vi "FP_Size Inside Bounds.vi"(7 "Work Space":T1, 8 "Error":errorcluster, 11 "VI Ref":refnum<vi>) -> (0 "Error Out":errorcluster, 1 "Vertical In Range Out":bool, 2 "Horizontal In Range Out":bool, 3 "VI Ref Out":refnum<vi>)   [LabVIEW 2016]
uses:
  <vilib>/Utility/miscctls.llb/LVRectTypeDef.ctl
panel:
  out "Front Panel Window:Window Bounds":T1
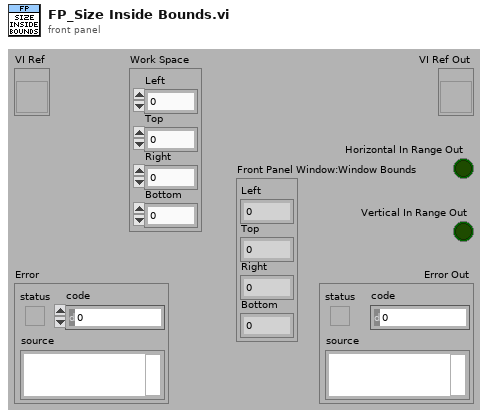
[diagram p1: front panel]
types:
  T1 = typedef "LVRectTypeDef.ctl" = cluster{"Left":i16, "Top":i16, "Right":i16, "Bottom":i16}
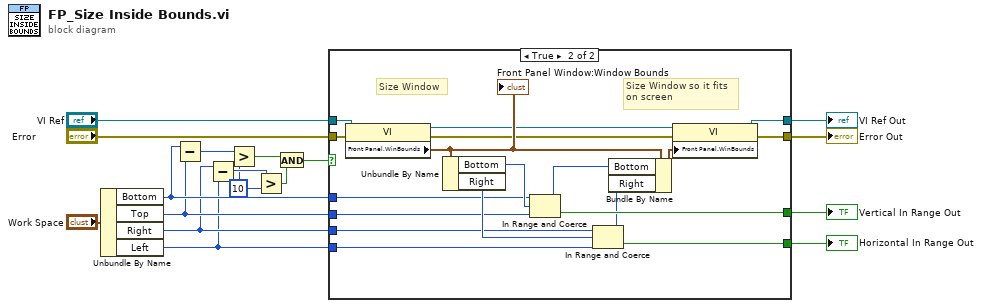
[diagram p0: block diagram]
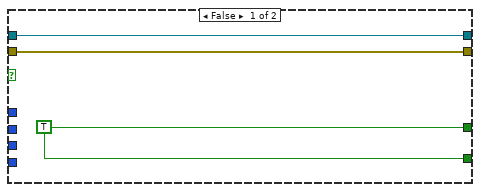
[diagram p2: hidden frame]
diagram:
  w4 = i16 10 ("y")
  n1 = Unbundle By Name("Work Space") -> ("Bottom"=w10:i16, "Top"=w9:i16, "Right"=w8:i16, "Left"=w7:i16)
  n2 = Subtract(x=w10, y=w9) -> (x-y=w6:i16)
  n3 = Subtract(x=w8, y=w7) -> (x-y=w5:i16)
  n4 = Greater?(x=w6, y=w4) -> (0:w2:bool)
  n5 = Greater?(x=w5, y=w4) -> (0:w3:bool)
  n6 = And(x=w2, y=w3) -> (x .and. y?=w1:bool)
  n7 = case shown="True" w1 {
    tunnel: [w18 w38] -> w17
    tunnel: [w18 w37] -> w16
    tunnel: [w20 w36] -> w15
    tunnel: [w19 w35] -> w14
    tunnel: "Error" -> [w19 w26]
    tunnel: "VI Ref" -> [w20 w25]
    tunnel: w10 -> [_ w24]
    tunnel: w9 -> [_ w23]
    tunnel: w8 -> [_ w22]
    tunnel: w7 -> [_ w21]
    frame False {
      w18 = TRUE
    }
    frame True {
      # "Size Window so it fits\non screen"
      # "Size Window"
      n8 = property class="VI"(reference=w25, error in=w26) -> (reference out=w27:refnum<vi>, error out=w28:errorcluster, "Front Panel.WinBounds"=w29:T1)
      "Front Panel Window:Window Bounds" <- w29
      n9 = Unbundle By Name(w29) -> ("Bottom"=w31:i16, "Right"=w33:i16)
      n10 = In Range and Coerce(upper limit=w24, x=w31, lower limit=w23) -> (coerced(x)=w32:i16, In Range?=w38:bool)
      n11 = In Range and Coerce(upper limit=w22, x=w33, lower limit=w21) -> (coerced(x)=w34:i16, In Range?=w37:bool)
      n12 = Bundle By Name(cluster=w29, "Bottom"=w32, "Right"=w34) -> (w30:T1)
      n13 = property class="VI"(reference=w27, error in=w28, "Front Panel.WinBounds"=w30) -> (reference out=w36:refnum<vi>, error out=w35:errorcluster)
    }
  }
  "Vertical In Range Out" <- w17
  "Horizontal In Range Out" <- w16
  "VI Ref Out" <- w15
  "Error Out" <- w14
